vi "FRIC_SF2_Get_NextState_ProcessLoop.vi"(11 "SF2 Process Loop TypeDef (in)":T1={"State Array"=[enum."Hault", enum."Process"], "error"={"status"=FALSE, "code"=0, "source"=""}, "SF2 Buffer"=[], "Loop Frequency"=200, "Buffer Size"=0.0, "notifier ref out"=refnum, "Sample rate"=200} {"Buffer Size" format="%#_6f"}) -> (3 "SF2 Process Loop TypeDef (out)":T1={"State Array"=[enum."Hault", enum."Process"], "error"={"status"=FALSE, "code"=0, "source"=""}, "SF2 Buffer"=[], "Loop Frequency"=200, "Buffer Size"=0.0, "notifier ref out"=refnum, "Sample rate"=200} {"Buffer Size" format="%#_6f"}, 5 "Current State":T2)   [LabVIEW 2016]
uses:
  FRIC_SF2_Process Loop TypeDef.ctl
  FRIC_SF2_ProcessingLoopStatesTypeDef_I2C.ctl
  _Notifier/SF2_NotifyPacketTypeDef.ctl
  _Notifier/SF2_ActionTypeDef.ctl
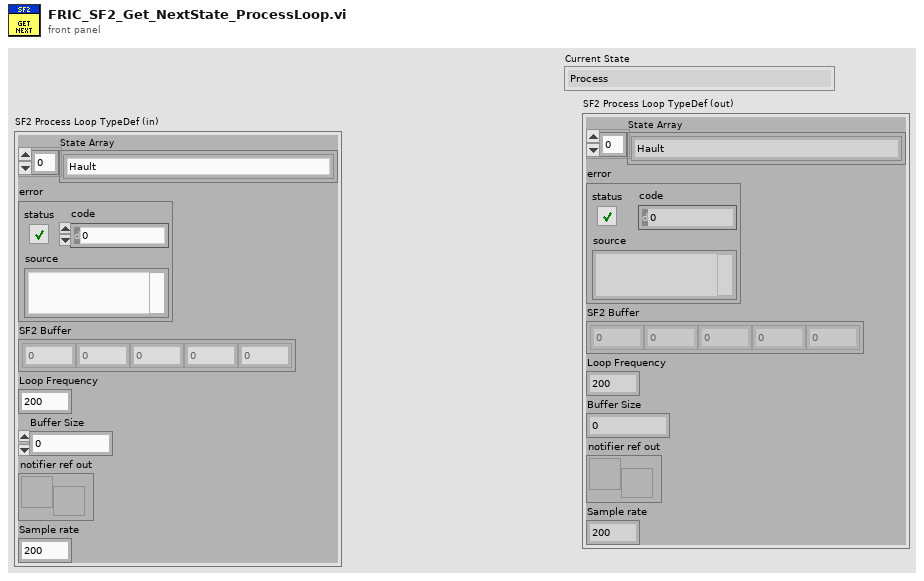
[diagram p1: front panel]
types:
  T1 = typedef "FRIC_SF2_Process Loop TypeDef.ctl" = cluster{"State Array":T2[], "error":errorcluster, "SF2 Buffer":dbl[][], "Loop Frequency":u32, "Buffer Size":dbl, "notifier ref out":refnum<notifier>, "Sample rate":u8}
  T2 = typedef "FRIC_SF2_ProcessingLoopStatesTypeDef_I2C.ctl" = enum16{"Process", "Hault", "Exit", "VI_INI"}
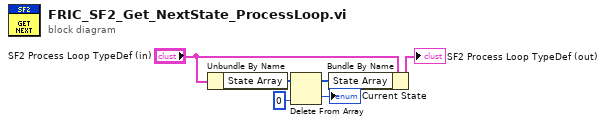
[diagram p0: block diagram]
diagram:
  n1 = Unbundle By Name("SF2 Process Loop TypeDef (in)") -> ("State Array"=w5:T2[])
  n2 = Delete From Array(array=w5, index=0) -> (deleted portion=→"Current State":T2, array with subset deleted=w3:T2[])  [unwired: 1 in]
  n3 = Bundle By Name(cluster="SF2 Process Loop TypeDef (in)", "State Array"=w3) -> (→"SF2 Process Loop TypeDef (out)":T1)
